vi "lockin - zero amplitude.vi"(6 "measure\noffset?":bool, 8 "error in (no error)":errorcluster, 11 "Lockin.DAQ":refnum<class "Lockin.DAQ.lvclass">) -> (0 "error out":errorcluster, 3 "Lockin.DAQ out":refnum<class "Lockin.DAQ.lvclass">)   [LabVIEW 2016, in "Lockin.DAQ.lvclass"]
uses:
  Lockin.DAQ.lvclass
  Lockin.DAQ.lvclass/Lockin.DAQ.ctl
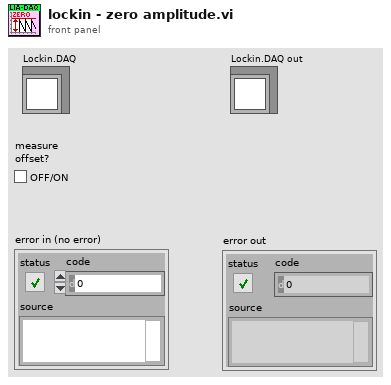
[diagram p1: front panel]
types:
  T1 = typedef "Lockin.DAQ.lvclass/AO-cluster.ctl" = T2[]
  T2 = typedef "Instrument.Lockin.UI.lvclass/AO Channel--Cluster.ctl" = cluster{"Channel":i32, "Amplitude":dbl, "Offset":dbl, "Frequency":dbl, "Phase":dbl, "Function":T3, "Sweeping?":bool, "REF.Ch 1":u16, "REF.Ch 2":u16}
  T3 = typedef "Lockin.DAQ.lvclass/Function-enum.ctl" = enum16{"Sine", "Triangle", "Square"}
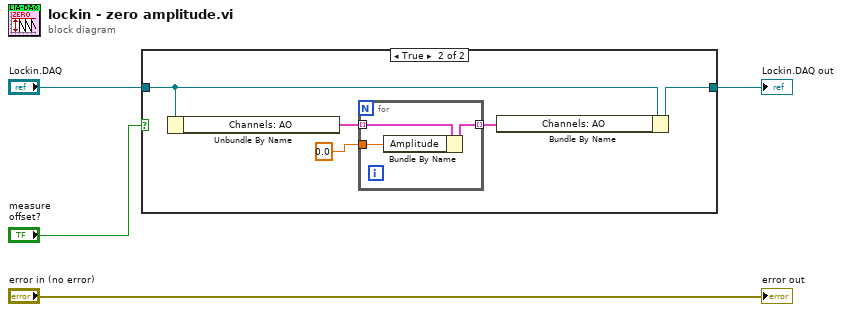
[diagram p0: block diagram]
diagram:
  n1 = case shown="True" "measure\noffset?" {
    tunnel: "Lockin.DAQ" -> [w5 w10]
    tunnel: [w5 w6] -> w2
    frame False {
    }
    frame True {
      n2 = Unbundle By Name(w10) -> ("Channels: AO"=w9:T1)
      n3 = for {
        tunnel: w9 -> [w12] mode=indexing
        tunnel: 0.0 ("element") -> [w13]
        tunnel: [w11] -> w7 mode=indexing
        n4 = Bundle By Name(cluster=w12, "Amplitude"=w13) -> (w11:T2)
      }
      n5 = Bundle By Name(cluster=w10, "Channels: AO"=w7) -> (w6:refnum<class "Lockin.DAQ.lvclass">)
    }
  }
  "Lockin.DAQ out" <- w2
  "error out" <- "error in (no error)"
